vi "Pixel Test.vi"(4 "Factor":dbl=1.0, 6 "Brightness":u8=50 min=1 step=1, 7 "stop":bool, 8 "error in (no error)":errorcluster, 9 "Period (ms)":u32=500, 10 "Color":u32(colorbox)=16777215, 11 "Refnum in":refnum<k20>) -> (0 "error out":errorcluster, 3 "Refnum out":refnum<k20>)   [LabVIEW 2013]
panel:
  in  "Test Data":u32[](array[numeric])=[16777215, 0, 0, 0, 0, 0, 0, 0, 0, 0, 0, 0, 0, 0, 0, 0, 0, 0, 0, 0, 0, 0, 0, 0, 0, 0, 0, 0, 0, 0, 0, 0, 0, 0, 0, 0, 0, 0, 0, 0, 0, 0, 0, 0, 0, 0, 0, 0, 0, 0, 0, 0, 0, 0, 0, 0, 0, 0, 0, 0, 0, 0, 0, 0, 0, 0, 0, 0, 0, 0, 0, 0, 0, 0, 0, 0, 0, 0, 0, 0, 0, 0, 0, 0, 0, 0, 0, 0, 0, 0, 0, 0, 0, 0, 0, 0, 0, 0, 0, 0, 0, 0, 0, 0, 0, 0, 0, 0, 0, 0, 0, 0, 0, 0, 0, 0, 0, 0, 0, 0, 0, 0, 0, 0, 0, 0, 0, 0, 0, 0, 0, 0, 0, 0, 0, 0, 0, 0, 0, 0, 0, 0, 0, 0, 0, 0, 0, 0, 0, 0, 0, 0, 0, 0, 0, 0, 0, 0, 0, 0, 0, 0, 0, 0, 0, 0, 0, 0, 0, 0, 0, 0, 0, 0, 0, 0, 0, 0, 0, 0, 0, 0, 0, 0, 0, 0, 0, 0, 0, 0, 0, 0, 0, 0, 0, 0, 0, 0, 0, 0, 0, 0, 0, 0, 0, 0, 0, 0, 0, 0, 0, 0, 0, 0, 0, 0, 0, 0, 0, 0, 0, 0, 0, 0, 0, 0, 0, 0, 0, 0, 0, 0, 0, 0, 0, 0, 0, 0, 0, 0, 0, 0, 0, 0, 0, 0, 0, 0, 0, 0, 0, 0, 0, 0, 0, 0, 0, 0, 0, 0, 0, 0, 0, 0, 0, 0, 0, 0, 0, 0, 0, 0, 0, 0, 0, 0, 0, 0, 0, 0, 0, 0, 0, 0, 0, 0, 0, 0, 0, 0, 0, 0, 0, 0, 0, 0, 0, 0, 0, 0, 0, 0, 0, 0, 0, 0, 0, 0, 0, 0, 0, 0, 0, 0, 0, 0, 0, 0, 0, 0, 0, 0, 0, 0, 0, 0, 0, 0, 0, 0, 0, 0, 0, 0, 0, 0, 0, 0, 0, 0, 0, 0, 0, 0, 0, 0, 0, 0, 0, 0, 0, 0, 0, 0, 0, 0, 0, 0, 0, 0, 0, 0, 0, 0, 0, 0, 0, 0, 0, 0, 0, 0, 0, 0, 0, 0, 0, 0, 0, 0, 0, 0, 0, 0, 0, 0, 0, 0, 0, 0, 0, 0, 0, 0, 0, 0, 0, 0, 0, 0, 0, 0, 0, 0, 0, 0, 0, 0, 0, 0, 0, 0, 0, 0, 0, 0, 0, 0, 0, 0, 0, 0, 0, 0, 0, 0, 0, 0, 0, 0, 0, 0, 0, 0, 0, 0, 0, 0, 0, 0, 0, 0, 0, 0, 0, 0, 0, 0, 0, 0, 0, 0, 0, 0, 0, 0, 0, 0, 0, 0, 0, 0, 0, 0, 0, 0, 0, 0, 0, 0, 0, 0, 0, 0, 0, 0, 0, 0, 0, 0, 0, 0, 0, 0, 0, 0, 0, 0, 0, 0, 0, 0, 0, 0, 0, 0, 0, 0, 0, 0, 0, 0, 0, 0, 0, 0, 0, 0, 0, 0, 0, 0] format="%x"
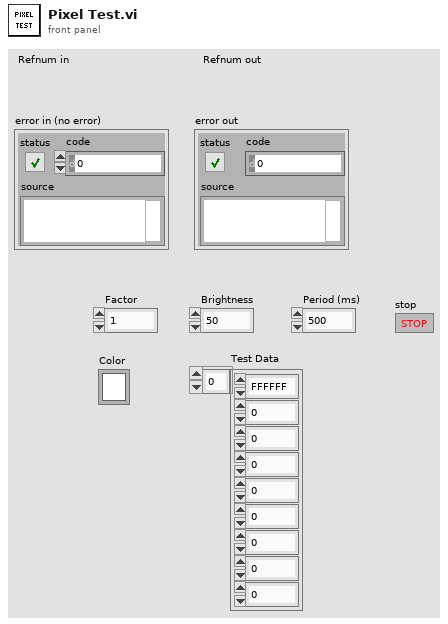
[diagram p1: front panel]
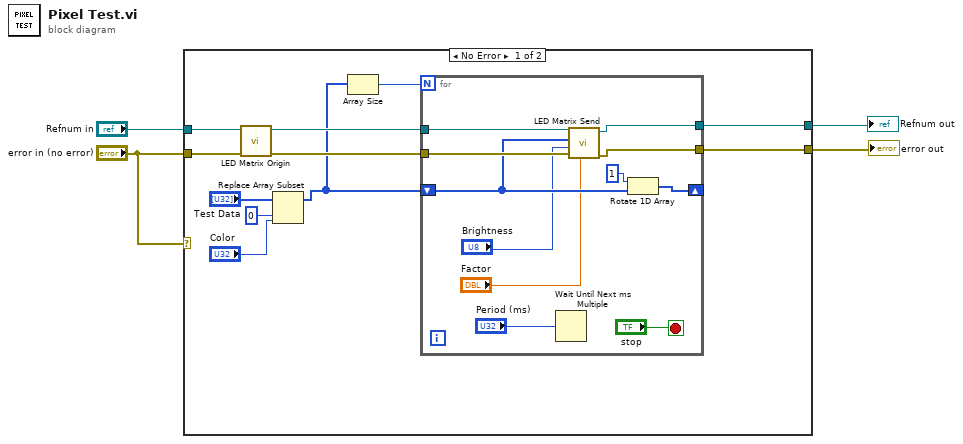
[diagram p0: block diagram]
diagram:
  n1 = case shown="No Error" "error in (no error)" {
    tunnel: "error in (no error)" -> [w12 w27]
    tunnel: "Refnum in" -> [w13 w28]
    tunnel: [w15 w28] -> w1
    tunnel: [w14 w27] -> w3
    frame No Error {
      n2 = call "LED Matrix Origin.vi"("error in (no error)"=w12, "Refnum in"=w13) -> ("error out"=w11:errorcluster, "Refnum out"=w10:refnum<k20>)  [unwired: 8 in]
      n3 = Replace Array Subset(array="Test Data", new element="Color", index=0) -> (w7:u32[])
      n4 = Array Size(array=w7) -> (size(s)=w9:i32)
      n5 = for {
        N: w9 -> [_]
        tunnel: [w26] -> w15
        tunnel: [w25] -> w14
        tunnel: w11 -> [w24]
        tunnel: w10 -> [w23]
        shift-right: [w20] -> _
        shift-left: w7 -> [w21]
        stop <- "stop" stop-if-true
        n6 = Wait Until Next ms Multiple(millisecond multiple="Period (ms)") -> ()  [unwired: 1 out]
        n7 = call "LED Matrix Send.vi"("Gamma"="Factor", "error in (no error)"=w24, "Brightness"="Brightness", "Data"=w21, "Refnum in"=w23) -> ("error out"=w25:errorcluster, "Refnum out"=w26:refnum<k20>)  [unwired: 3 in, 1 out]
        n8 = Rotate 1D Array(1:w21, 2:1 ("n")) -> (0:w20:u32[])
      }
    }
    frame Error {
    }
  }
  "error out" <- w3
  "Refnum out" <- w1
